vi "Microgear_onMessage.vi"(9 "lenght":u8, 10 "msg":string, 11 "topic":string) -> ()   [LabVIEW 2014]
uses:
  QwaveSys_ESP8266/QwaveSys_ESP8266.lvlib
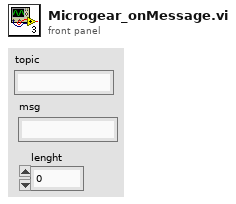
[diagram p1: front panel]
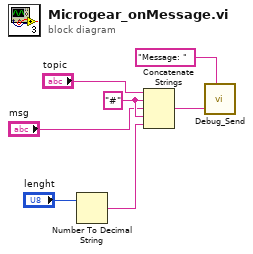
[diagram p0: block diagram]
diagram:
  w6 = "#" ("string")
  n1 = Number To Decimal String(number="lenght") -> (decimal integer string=w5:string)  [unwired: 1 in]
  n2 = Concatenate Strings("topic", w6, "msg", w6, w5) -> (w4:string)
  n3 = call "Debug_Send.vi"("Name"="Message: ", "DATA"=w4) -> ()  [unwired: 10 in]
